vi "CreateTextFile.vi"(11 "Input File Path":path) -> ()   [LabVIEW 2019, in "FileUtilities.lvlib"]
uses:
  FileUtilities.lvlib
  Modules/ModuleB/ModuleStatus.ctl
  Modules/ModuleB/ModuleB.lvlib
panel:
  in  "Module Status":T1
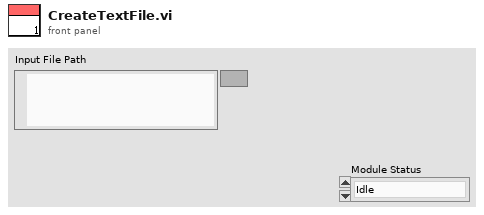
[diagram p1: front panel]
types:
  T1 = typedef "ModuleB.lvlib/ModuleStatus.ctl" = enum16{"Idle", "Running"}
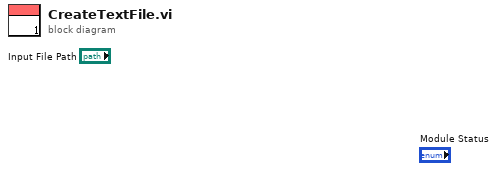
[diagram p0: block diagram]
diagram:
